vi "Init Data.vi"(10 "Data":T1) -> (3 "Msg out":refnum<class "Msg.lvclass">)   [LabVIEW 2020, in "CmdDigitalMultiple.lvlib" / "Msg.lvclass"]
uses:
  Msg.lvclass
  Data.ctl
  CmdDigital/Data.ctl
  Msg.lvclass/Msg.ctl
  CmdDigitalMultiple.lvlib
  CmdDigital/CmdDigital.lvlib
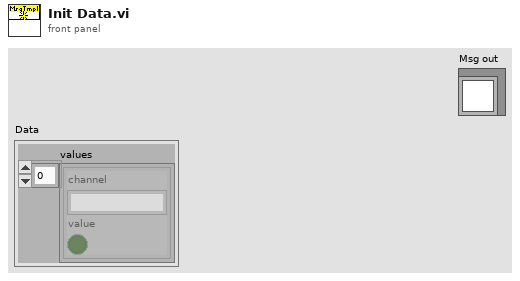
[diagram p1: front panel]
types:
  T1 = typedef "CmdDigitalMultiple.lvlib/Data.ctl" = cluster{"values":T2[]}
  T2 = typedef "CmdDigital.lvlib/Data.ctl" = cluster{"channel":string, "value":bool}
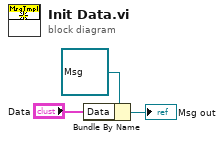
[diagram p0: block diagram]
diagram:
  n1 = Bundle By Name(cluster=refnum<class "Msg.lvclass"> refnum ("Msg out"), "Data"="Data") -> (→"Msg out":refnum<class "Msg.lvclass">)
